vi "Write Data.vi"(7 "TX.Data":T1 caption="Transmission Data" format="%.0x", 8 "error in (no error)":errorcluster, 11 "Low Speed in":refnum<class "Low Speed.lvclass">) -> (0 "error out":errorcluster, 3 "Low Speed out":refnum<class "Low Speed.lvclass">)   [LabVIEW 2020, in "Low Speed.lvclass"]
uses:
  Low Speed.lvclass
  C:/Users/kaiser.asan/OneDrive - SolitonTechnologies/LabVIEW/29.SDLC - I2C Driver/I2C Module/I2C Controller Module/Class/Transmission Mode/Parent/TX Speed.lvclass
  TypeDef/Transmission Data.ctl
  Parent/TX Speed.lvclass
  I2C Controller Lib.lvlib
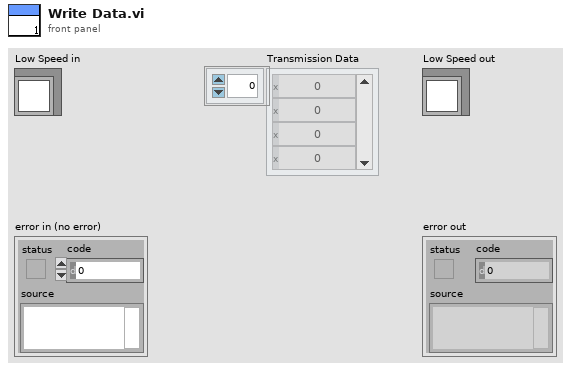
[diagram p1: front panel]
types:
  T1 = typedef "I2C Controller Lib.lvlib/Transmission Data.ctl" = u8[]
  T2 = typedef "I2C Controller Lib.lvlib/Timing Parameters Cluster.ctl" = cluster{"f_SCL(KHz)":u32, "t_HIGH (ns)":u32, "t_LOW (ns)":u32, "t_SU;STA (ns)":u32, "t_HD;STA (ns)":u32, "t_SU;DAT (ns)":u32, "t_HD;DAT (ns)":u32, "t_SU;STO (ns)":u32, "t_BUF (ns)":u32}
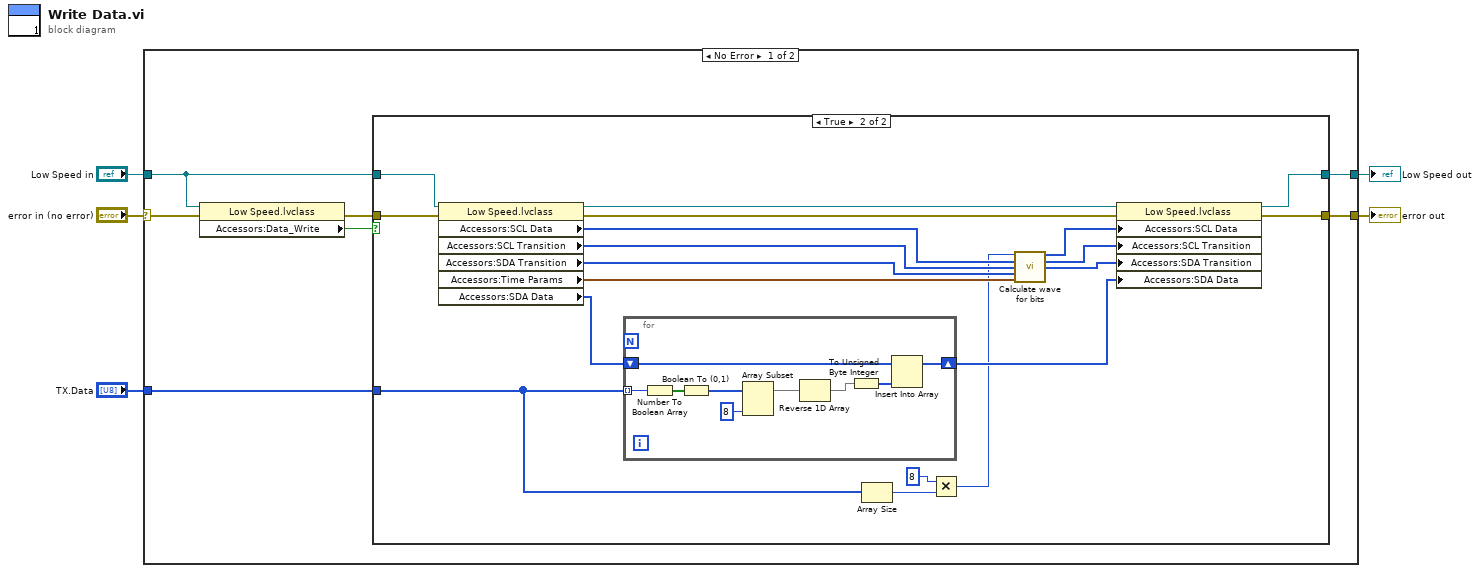
[diagram p0: block diagram]
diagram:
  n1 = case shown="No Error" "error in (no error)" {
    selector: "error in (no error)" -> [w12 w44]
    tunnel: [w11 w44] -> w5
    tunnel: [w9 w43] -> w3
    tunnel: "Low Speed in" -> [w8 w43]
    tunnel: "TX.Data" -> [w6 _]
    frame No Error {
      n2 = property class="Low Speed.lvclass"(reference=w8, error in=w12) -> (error out=w10:errorcluster, "Accessors:Data_Write"=w7:bool)  [unwired: 1 out]
      n3 = case shown="True" w7 {
        tunnel: [w13 w31] -> w11
        tunnel: w10 -> [w13 w33]
        tunnel: [w14 w29] -> w9
        tunnel: w8 -> [w14 w28]
        tunnel: w6 -> [_ w18]
        frame False {
        }
        frame True {
          n4 = property class="Low Speed.lvclass"(reference=w28, error in=w33) -> (reference out=w30:refnum<class "Low Speed.lvclass">, error out=w32:errorcluster, "Accessors:SCL Data"=w27:u8[], "Accessors:SCL Transition"=w26:u32[], "Accessors:SDA Transition"=w25:u32[], "Accessors:Time Params"=w24:T2, "Accessors:SDA Data"=w20:u8[])
          n5 = for {
            tunnel: w18 -> [w38] mode=indexing
            shift-right: [w35] -> w19
            shift-left: w20 -> [w34]
            n6 = Number To Boolean Array(number=w38) -> (Boolean array=w42:bool[])
            n7 = Boolean To (0,1)(Boolean=w42) -> (0, 1=w41:i16[])
            n8 = Array Subset(array=w41, length=8) -> (w40:i16[])  [unwired: 1 in]
            n9 = Reverse 1D Array(array=w40) -> (reversed array=w37:i16[])
            n10 = To Unsigned Byte Integer(number=w37) -> (unsigned 8bit integer=w36:u8[])
            n11 = Insert Into Array(array=w34, new element=w36) -> (w35:u8[])  [unwired: 1 in]
          }
          n12 = Array Size(array=w18) -> (size(s)=w17:i32)
          n13 = Multiply(x=8, y=w17) -> (x*y=w15:i32)
          n14 = call "Calculate wave for bits.vi"("No. Of Bits"=w15, "SCL DATA IN"=w27, "SCL Transitions In"=w26, "SDA Transitions In"=w25, "Time Params"=w24) -> ("SCL DATA OUT"=w23:u8[], "SCL Transitions Out"=w22:u32[], "SDA Transitions Out"=w21:u32[])  [unwired: 8 in]
          n15 = property class="Low Speed.lvclass"(reference=w30, error in=w32, "Accessors:SCL Data"=w23, "Accessors:SCL Transition"=w22, "Accessors:SDA Transition"=w21, "Accessors:SDA Data"=w19) -> (reference out=w29:refnum<class "Low Speed.lvclass">, error out=w31:errorcluster)
        }
      }
    }
    frame Error {
    }
  }
  "error out" <- w5
  "Low Speed out" <- w3
